vi "String to Variant.vi"(7 "Value Type":T1, 11 "String":string) -> (2 "error out":errorcluster, 3 "Variant":variant, 5 "Invalid Format":bool)   [LabVIEW 2020, in "Parallel Block.lvlib"]
uses:
  Parallel Block.lvlib
  Value Type.ctl
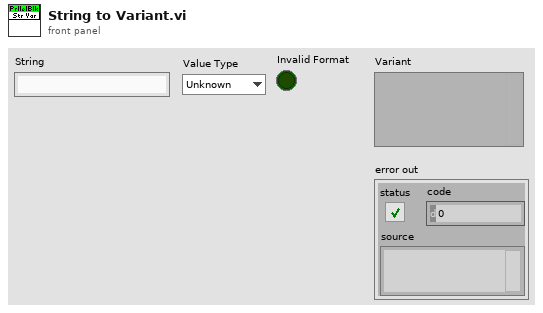
[diagram p1: front panel]
types:
  T1 = typedef "Parallel Block.lvlib/Value Type.ctl" = enum16{"Unknown", "Bool", "U8", "U16", "U32", "U64", "I8", "I16", "I32", "I64", "SGL", "DBL", "CSG", "CDB", "CDBWfm", "String", "DBLWfm"}
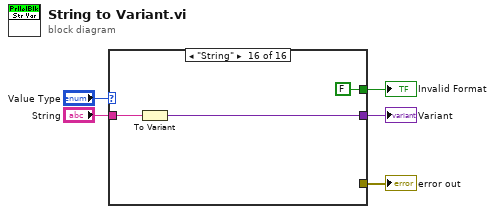
[diagram p0: block diagram]
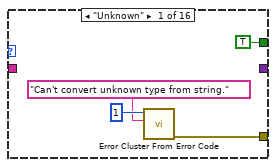
[diagram p2: hidden frame]
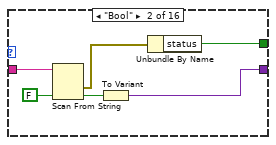
[diagram p3: hidden frame]
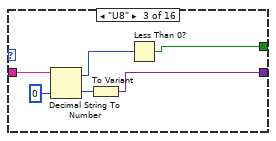
[diagram p4: hidden frame]
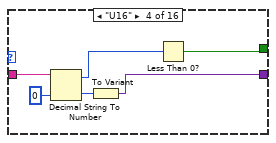
[diagram p5: hidden frame]
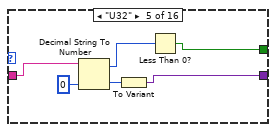
[diagram p6: hidden frame]
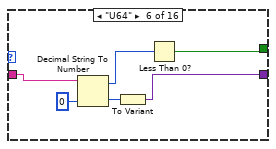
[diagram p7: hidden frame]
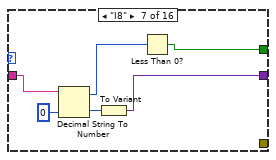
[diagram p8: hidden frame]
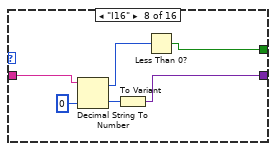
[diagram p9: hidden frame]
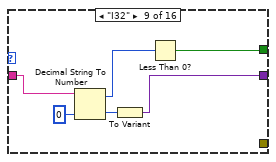
[diagram p10: hidden frame]
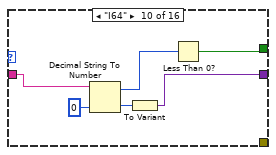
[diagram p11: hidden frame]
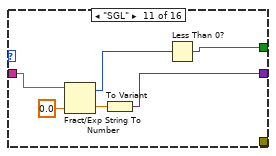
[diagram p12: hidden frame]
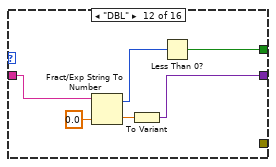
[diagram p13: hidden frame]
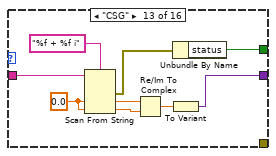
[diagram p14: hidden frame]
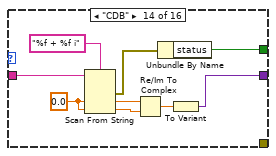
[diagram p15: hidden frame]
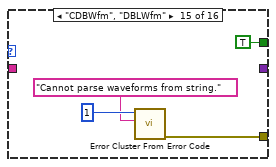
[diagram p16: hidden frame]
diagram:
  n1 = case shown="\"String\"" "Value Type" {
    tunnel: "String" -> [_ w15 w21 w25 w31 w37 w43 w49 w55 w61 w67 w73 w84 w93 _ w100]
    tunnel: [_ w12 w18 w24 w30 w36 w42 w48 w54 w60 w66 w72 w78 w87 _ w99] -> w3
    tunnel: [w7 _ _ _ _ _ _ _ _ _ _ _ _ _ w95 _] -> w2
    tunnel: [TRUE ("status") w10 w16 w22 w28 w34 w40 w46 w52 w58 w64 w70 w76 w85 TRUE ("status") FALSE ("status")] -> w1
    frame "Unknown" {
      n2 = call <vilib>:"Error Cluster From Error Code.vi"("error message (\"\")"="Can't convert unknown type from string." ("error message (\"\")"), "error code (0)"=1) -> ("error out"=w7:errorcluster)  [unwired: 7 in]
    }
    frame "Bool" {
      n3 = Scan From String(input string=w15, default 1=FALSE) -> (error out=w11:errorcluster, output 1=w13:bool)  [unwired: 3 in, 2 out]
      n4 = To Variant(anything=w13) -> (Variant=w12:variant)
      n5 = Unbundle By Name(w11) -> ("status"=w10:bool)
    }
    frame "U8" {
      n6 = Decimal String To Number(string=w21, default (0L)=u8 0 ("default (0 I32)")) -> (offset past number=w17:i32, number=w19:u8)  [unwired: 1 in]
      n7 = To Variant(anything=w19) -> (Variant=w18:variant)
      n8 = Less Than 0?(x=w17) -> (x < 0?=w16:bool)
    }
    frame "U16" {
      n9 = Decimal String To Number(string=w25, default (0L)=u16 0 ("default (0 I32)")) -> (offset past number=w23:i32, number=w26:u16)  [unwired: 1 in]
      n10 = To Variant(anything=w26) -> (Variant=w24:variant)
      n11 = Less Than 0?(x=w23) -> (x < 0?=w22:bool)
    }
    frame "U32" {
      n12 = Decimal String To Number(string=w31, default (0L)=u32 0 ("default (0 I32)")) -> (offset past number=w29:i32, number=w32:u32)  [unwired: 1 in]
      n13 = To Variant(anything=w32) -> (Variant=w30:variant)
      n14 = Less Than 0?(x=w29) -> (x < 0?=w28:bool)
    }
    frame "U64" {
      n15 = Decimal String To Number(string=w37, default (0L)=u64 0 ("default (0 I32)")) -> (offset past number=w35:i32, number=w38:u64)  [unwired: 1 in]
      n16 = To Variant(anything=w38) -> (Variant=w36:variant)
      n17 = Less Than 0?(x=w35) -> (x < 0?=w34:bool)
    }
    frame "I8" {
      n18 = Decimal String To Number(string=w43, default (0L)=i8 0 ("default (0 I32)")) -> (offset past number=w41:i32, number=w44:i8)  [unwired: 1 in]
      n19 = To Variant(anything=w44) -> (Variant=w42:variant)
      n20 = Less Than 0?(x=w41) -> (x < 0?=w40:bool)
    }
    frame "I16" {
      n21 = Decimal String To Number(string=w49, default (0L)=i16 0 ("default (0 I32)")) -> (offset past number=w47:i32, number=w50:i16)  [unwired: 1 in]
      n22 = To Variant(anything=w50) -> (Variant=w48:variant)
      n23 = Less Than 0?(x=w47) -> (x < 0?=w46:bool)
    }
    frame "I32" {
      n24 = Decimal String To Number(string=w55, default (0L)=0 ("default (0 I32)")) -> (offset past number=w53:i32, number=w56:i32)  [unwired: 1 in]
      n25 = To Variant(anything=w56) -> (Variant=w54:variant)
      n26 = Less Than 0?(x=w53) -> (x < 0?=w52:bool)
    }
    frame "I64" {
      n27 = Decimal String To Number(string=w61, default (0L)=i64 0 ("default (0 I32)")) -> (offset past number=w59:i32, number=w62:i64)  [unwired: 1 in]
      n28 = To Variant(anything=w62) -> (Variant=w60:variant)
      n29 = Less Than 0?(x=w59) -> (x < 0?=w58:bool)
    }
    frame "SGL" {
      n30 = Fract/Exp String To Number(string=w67, default (0 dbl)=sgl 0.0 ("default (0 I32)")) -> (offset past number=w65:i32, number=w68:sgl)  [unwired: 2 in]
      n31 = To Variant(anything=w68) -> (Variant=w66:variant)
      n32 = Less Than 0?(x=w65) -> (x < 0?=w64:bool)
    }
    frame "DBL" {
      n33 = Fract/Exp String To Number(string=w73, default (0 dbl)=sgl 0.0 ("default (0 I32)")) -> (offset past number=w71:i32, number=w74:sgl)  [unwired: 2 in]
      n34 = To Variant(anything=w74) -> (Variant=w72:variant)
      n35 = Less Than 0?(x=w71) -> (x < 0?=w70:bool)
    }
    frame "CSG" {
      w82 = sgl 0.0 ("default value 1")
      n36 = Scan From String(format string="%f + %f i", input string=w84, default 1=w82, default 2=w82) -> (error out=w77:errorcluster, output 1=w81:sgl, output 2=w80:sgl)  [unwired: 2 in, 2 out]
      n37 = Re/Im To Complex(1:w80, 2:w81) -> (0:w79:csg)
      n38 = To Variant(anything=w79) -> (Variant=w78:variant)
      n39 = Unbundle By Name(w77) -> ("status"=w76:bool)
    }
    frame "CDB" {
      w91 = 0.0 ("default value 1")
      n40 = Scan From String(format string="%f + %f i", input string=w93, default 1=w91, default 2=w91) -> (error out=w86:errorcluster, output 1=w90:dbl, output 2=w89:dbl)  [unwired: 2 in, 2 out]
      n41 = Re/Im To Complex(1:w89, 2:w90) -> (0:w88:cdb)
      n42 = Unbundle By Name(w86) -> ("status"=w85:bool)
      n43 = To Variant(anything=w88) -> (Variant=w87:variant)
    }
    frame "CDBWfm", "DBLWfm" {
      n44 = call <vilib>:"Error Cluster From Error Code.vi"("error message (\"\")"="Cannot parse waveforms from string." ("error message (\"\")"), "error code (0)"=1) -> ("error out"=w95:errorcluster)  [unwired: 7 in]
    }
    frame "String" {
      n45 = To Variant(anything=w100) -> (Variant=w99:variant)
    }
  }
  "Variant" <- w3
  "error out" <- w2
  "Invalid Format" <- w1
